vi "Pre Launch Init.vi"(11 "Simulated Wash Display Console Actor in":refnum<class "Simulated Wash Display Console Actor.lvclass">) -> (0 "error out":errorcluster, 3 "Simulated Wash Display Console Actor out":refnum<class "Simulated Wash Display Console Actor.lvclass">)   [LabVIEW 2019, in "Simulated Wash Display Console Actor.lvlib" / "Simulated Wash Display Console Actor.lvclass"]
doc: "(<B>Filename</B>: Actor Framework.lvlib:Actor.lvclass:Pre Launch Init.vi)\n\nDefines behavior that occurs after the Launch Nested Actor method is invoked but before the actor's Actor Core method begins running.\n\nBy default, this method does nothing. A descendant class may override it to define behavior."
uses:
  Simulated Wash Display Console Actor.lvclass
  Simulated Wash Display Console Actor.lvclass/Simulated Wash Display Console Actor.ctl
  Abstract Washer Display Console Actor/Abstract Washer Display Console Actor/Washer Display Console Actor.lvclass
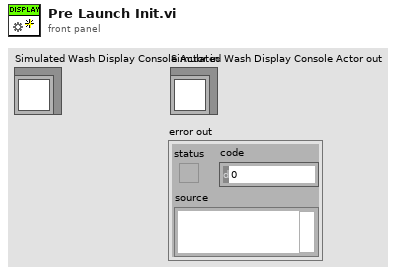
[diagram p1: front panel]
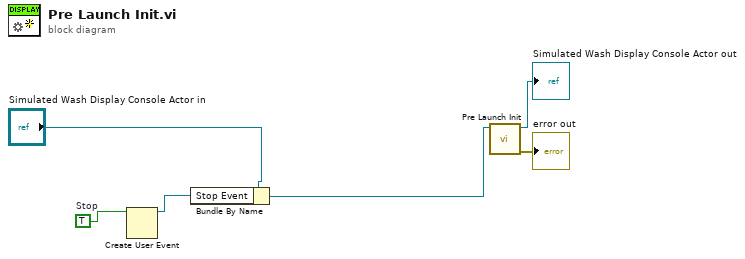
[diagram p0: block diagram]
diagram:
  w3 = TRUE  # Stop
  n1 = Create User Event(user event datatype=w3) -> (user event=w4:refnum<user-event>)  [unwired: 1 in, 1 out]
  n2 = Bundle By Name(cluster="Simulated Wash Display Console Actor in", "Stop Event"=w4) -> (w1:refnum<class "Simulated Wash Display Console Actor.lvclass">)
  n3 = call-parent "Pre Launch Init.vi"("Actor in"=w1) -> ("error out"=→"error out":errorcluster, "Actor out"=→"Simulated Wash Display Console Actor out":refnum<class "Simulated Wash Display Console Actor.lvclass">)  [unwired: 9 in]
